vi "Shutdown1287.vi"(6 "Error In (No Error)":errorcluster, 9 "VISA Name In":refnum<visa-resource-name>="Solartron1287") -> (0 "error out":errorcluster, 3 "VISA resource name out":refnum<visa-resource-name>)   [LabVIEW 2018]
panel:
  # "Standalone VI for shutting down 1287 Potentiostat"
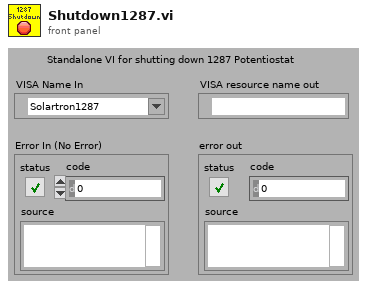
[diagram p1: front panel]
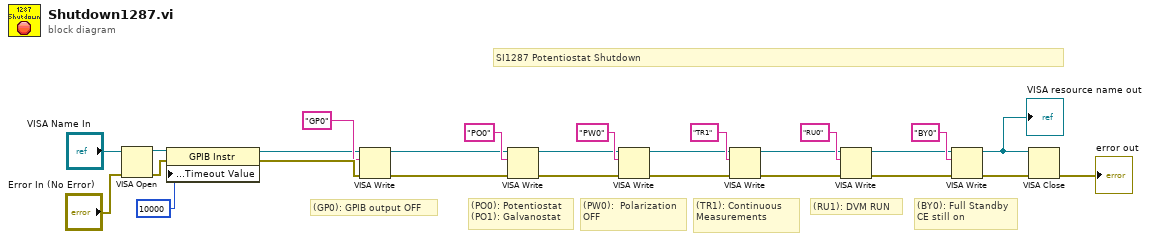
[diagram p0: block diagram]
diagram:
  # "(GP0): GPIB output OFF"
  # "(BY0): Full Standby\nCE still on"
  # "(RU1): DVM RUN"
  # "(TR1): Continuous Measurements"
  # "(PW0):  Polarization OFF"
  # "(PO0): Potentiostat\n(PO1): Galvanostat"
  # "SI1287 Potentiostat Shutdown"
  n1 = VISA Open(error in (no error)="Error In (No Error)", VISA resource name="VISA Name In") -> (VISA resource name=w7:refnum<visa-resource-name>, error out=w6:errorcluster)  [unwired: 3 in]
  n2 = property class="GPIB Instr"(reference=w7, error in=w6, "General Settings:Timeout Value"=u32 10000) -> (reference out=w1:refnum<visa-resource-name>, error out=w3:errorcluster)
  n3 = VISA Write(VISA resource name=w1, write buffer="GP0" ("Characters to Write"), error in (no error)=w3) -> (VISA resource name out=w5:refnum<visa-resource-name>, error out=w4:errorcluster)  [unwired: 1 out]
  n4 = VISA Write(VISA resource name=w5, write buffer="PO0", error in (no error)=w4) -> (VISA resource name out=w21:refnum<visa-resource-name>, error out=w17:errorcluster)  [unwired: 1 out]
  n5 = VISA Write(VISA resource name=w21, write buffer="PW0", error in (no error)=w17) -> (VISA resource name out=w20:refnum<visa-resource-name>, error out=w16:errorcluster)  [unwired: 1 out]
  n6 = VISA Write(VISA resource name=w20, write buffer="TR1", error in (no error)=w16) -> (VISA resource name out=w19:refnum<visa-resource-name>, error out=w15:errorcluster)  [unwired: 1 out]
  n7 = VISA Write(VISA resource name=w19, write buffer="RU0", error in (no error)=w15) -> (VISA resource name out=w18:refnum<visa-resource-name>, error out=w14:errorcluster)  [unwired: 1 out]
  n8 = VISA Write(VISA resource name=w18, write buffer="BY0", error in (no error)=w14) -> (VISA resource name out=w12:refnum<visa-resource-name>, error out=w13:errorcluster)  [unwired: 1 out]
  "VISA resource name out" <- w12
  n9 = VISA Close(VISA resource name=w12, error in (no error)=w13) -> (error out=→"error out":errorcluster)
